vi "_incrementHeadIndex.vi"(10 "NbElements":i32=1, 11 "VariantBuffer in":refnum<class "VariantBuffer.lvclass">) -> (3 "VariantBuffer out":refnum<class "VariantBuffer.lvclass">)   [LabVIEW 2013, in "CircularBuffer.lvlib" / "VariantBuffer.lvclass"]
uses:
  VariantBuffer.lvclass
  VariantBuffer.lvclass/VariantBuffer.ctl
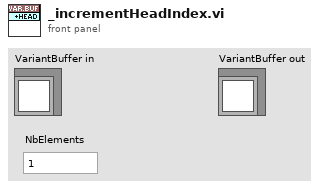
[diagram p1: front panel]
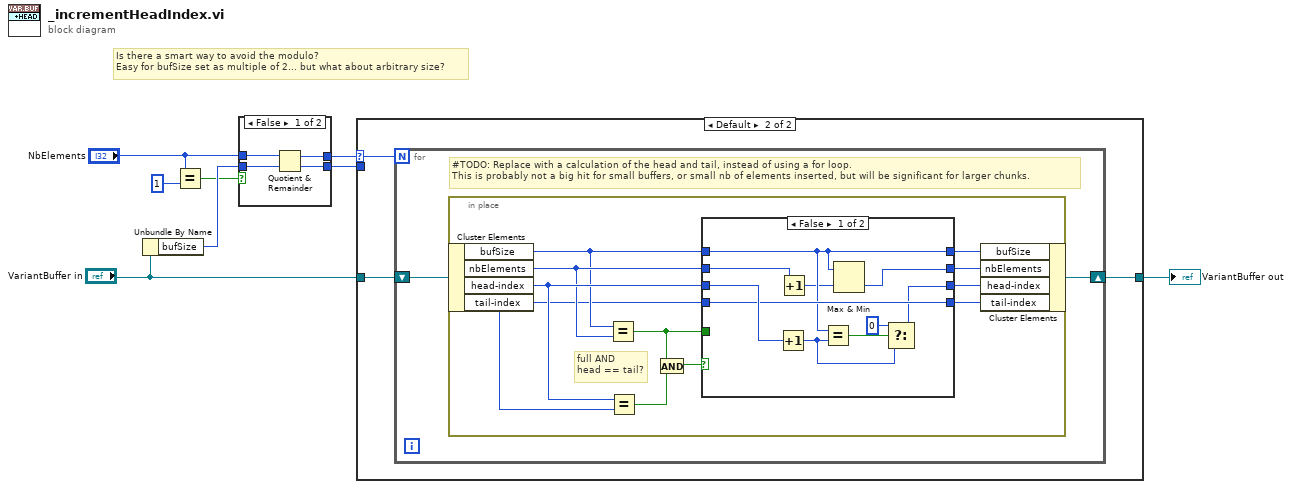
[diagram p0: block diagram]
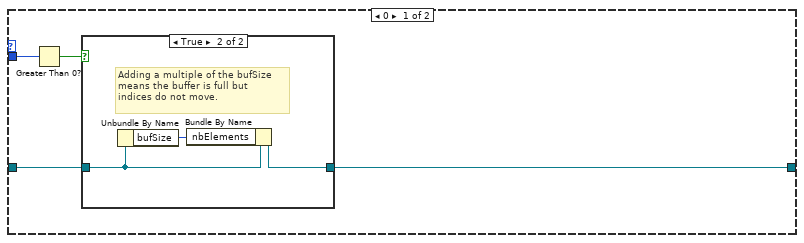
[diagram p3: hidden frame]
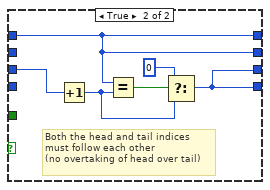
[diagram p5: hidden frame]
diagram:
  # "Is there a smart way to avoid the modulo?\nEasy for bufSize set as multiple of 2... but what about arbitrary size?"
  n1 = Unbundle By Name("VariantBuffer in") -> ("bufSize"=w6:i32)
  n2 = Equal?(x="NbElements", y=1) -> (x = y?=w1:bool)
  n3 = case shown="False" w1 {
    tunnel: w6 -> [w12 _]
    tunnel: [w11 w13] -> w5
    tunnel: [w10 _] -> w4
    tunnel: "NbElements" -> [w9 w13]
    frame False {
      n4 = Quotient & Remainder(x=w9, y=w12) -> (x-y*floor(x/y)=w11:i32, floor(x/y)=w10:i32)
    }
    frame True {
      # "1"
    }
  }
  n5 = case shown="Default" w5 {
    selector: w5 -> [_ w22]
    tunnel: [w16 w24] -> w8
    tunnel: "VariantBuffer in" -> [w15 w23]
    tunnel: w4 -> [w17 _]
    frame 0 {
      n6 = Greater Than 0?(x=w17) -> (x > 0?=w14:bool)
      n7 = case shown="True" w14 {
        tunnel: [w18 w20] -> w16
        tunnel: w15 -> [w18 w19]
        frame False {
          # "This case means we are moving by\nexactly 0 element."
        }
        frame True {
          # "Adding a multiple of the bufSize\nmeans the buffer is full but\nindices do not move."
          n8 = Unbundle By Name(w19) -> ("bufSize"=w21:i32)
          n9 = Bundle By Name(cluster=w19, "nbElements"=w21) -> (w20:refnum<class "VariantBuffer.lvclass">)
        }
      }
    }
    frame Default {
      n10 = for {
        N: w22 -> [_]
        shift-right: [w26] -> w24
        shift-left: w23 -> [w25]
        # "#TODO: Replace with a calculation of the head and tail, instead of using a for loop.\nThis is probably not a big hit for small buffers, or small nb of elements inserted, but will be significant for larger chunks."
        n11 = in-place {
          # "full AND\nhead == tail?"
          n12 = in-place-cluster #1(w25) -> ("bufSize"=w32:i32, "nbElements"=w34:i32, "head-index"=w35:i32, "tail-index"=w28:i32)
          n13 = Equal?(x=w32, y=w34) -> (x = y?=w27:bool)
          n14 = Equal?(x=w35, y=w28) -> (x = y?=w33:bool)
          n15 = And(x=w27, y=w33) -> (x .and. y?=w29:bool)
          n16 = case shown="False" w29 {
            tunnel: [w38 w48] -> w37
            tunnel: [w39 w52] -> w36
            tunnel: w35 -> [w45 w53]
            tunnel: w34 -> [w42 _]
            tunnel: w32 -> [w41 w52]
            tunnel: [w41 w52] -> w31
            tunnel: [w44 w48] -> w30
            tunnel: w28 -> [w44 _]
            tunnel: w27 -> [_ _]
            frame False {
              n17 = Increment(x=w45) -> (x+1=w46:i32)
              n18 = Increment(x=w42) -> (x+1=w40:i32)
              n19 = Equal?(x=w41, y=w46) -> (x = y?=w43:bool)
              n20 = Max & Min(x=w41, y=w40) -> (min(x,y)=w39:i32)  [unwired: 1 out]
              n21 = Select(t=0, s=w43, f=w46) -> (s? t:f=w38:i32)
            }
            frame True {
              # "Both the head and tail indices\nmust follow each other \n(no overtaking of head over tail)"
              n22 = Increment(x=w53) -> (x+1=w49:i32)
              n23 = Equal?(x=w52, y=w49) -> (x = y?=w51:bool)
              n24 = Select(t=0, s=w51, f=w49) -> (s? t:f=w48:i32)
            }
          }
          n25 = in-place-cluster #1("bufSize"=w31, "nbElements"=w36, "head-index"=w37, "tail-index"=w30) -> (w26:refnum<class "VariantBuffer.lvclass">)
        }
      }
    }
  }
  "VariantBuffer out" <- w8
